vi "UUT select.vi"(8 "error constant":errorcluster, 11 "UUT":u16(ring)=3 items=["BLDC 30A", "BLDC 60A", "Warrior 60A", "Condenser Merkava", "Condenser India"]) -> (0 "error constant 2":errorcluster, 2 "UUT Out":string, 3 "UUT Out":u16(ring)=3 items=["BLDC  30A  P/N: 500490", "BLDC  60A  P/N: 500390", "Warrior 60A P/N: 500590", "Condenser Merkava P/N: 5310003", "Condenser India P/N: 172774605"])   [LabVIEW 2017]
panel:
  in  "Next Button":bool
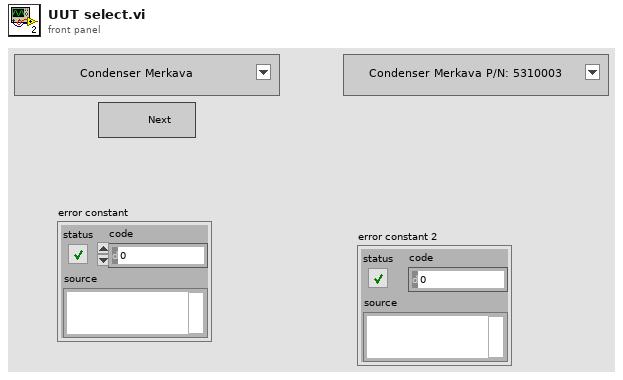
[diagram p1: front panel]
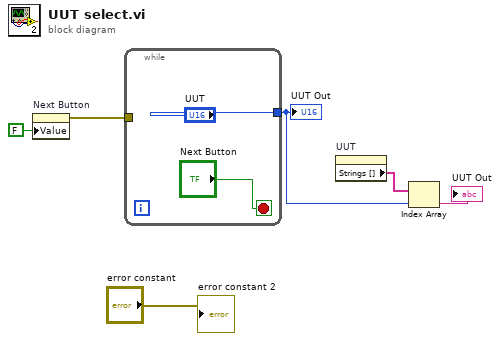
[diagram p0: block diagram]
diagram:
  n1 = property on="Next Button" class="Bool (strict)"("Value"=FALSE ("Next Button")) -> (error out=w4:errorcluster)  [unwired: 2 in, 1 out]
  n2 = while {
    tunnel: ["UUT"] -> w2
    tunnel: w4 -> [_]
    stop <- "Next Button" stop-if-true
  }
  "UUT Out" <- w2
  n3 = property on="UUT" class="Ring (strict)"() -> ("Strings []"=w3:string[])  [unwired: 2 in, 2 out]
  n4 = Index Array(array=w3, index=w2) -> (element=→"UUT Out":string)
  "error constant 2" <- "error constant"
